vi "dataListenerMain.vi"() -> ()   [LabVIEW 2016]
doc: "Starts the Data Listener application. This method is the the same for each component."
uses:
  DataListenerThisComponent/DataListenerThisComponent.lvclass
  home/andres/ct_cmpuserevents/ComponentTemplateCore/ComponentModel/ComponentModel/DataListener/DataListener.lvclass
  CommandFactory/CommandFactory.lvclass
  home/andres/ct_cmpuserevents/ICommandFactory/ICommandFactory.lvclass
  PubSubDataEvent/PubSubDataEvent.lvclass
  ComponentTemplateCore/ComponentModel/ComponentModel/CommandEvent/CommandEvent.lvclass
  ComponentTemplateCore/ComponentModel/ComponentModel/MiddlewareProcessEvent/MiddlewareProcessEvent.lvclass
  ComponentTemplateCore/ComponentModel/ComponentModel/Rendezvous/Rendezvous.lvclass
  MiddlewareSALThisComponent/MiddlewareSALThisComponent.lvclass
  home/andres/ct_cmpuserevents/ComponentTemplateCore/ComponentModel/ComponentModel/Middleware/Middleware.lvclass
  MiddlewareSALThisComponent/ProgrammaticInitialization/ProgrammaticInitialization.lvclass
  DataListenerThisComponent/DataListenerThisComponent.lvclass/DataListenerThisComponent.ctl
  ComponentTemplateCore/ComponentModel/ComponentModel/Middleware/Middleware.lvclass/Middleware.ctl
  ComponentTemplateCore/ComponentModel/ComponentModel/DataListener/DataListener.lvclass/DataListener.ctl
  ComponentTemplateCore/ComponentModel/ComponentModel/DataListener/DataListener.lvclass
  ComponentTemplateCore/ComponentModel/ComponentModel/Middleware/Middleware.lvclass
  ComponentTemplateCore/ComponentModel/ComponentModel/ConfigurationFileReader/ConfigurationFileReader.lvclass
panel:
  out "error out":errorcluster
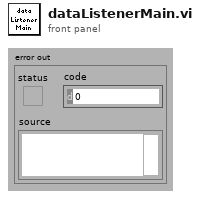
[diagram p1: front panel]
types:
  T1 = typedef "ConfigurationTypedefs.lvlib/SALVisSettings.ctl" = cluster{"SAL Vis Path":path, "Events":T2, "Telemetry":T3, "Subsystem":string, "Commands":T4}
  T2 = typedef "ProgrammaticInitialization.lvclass/evntsToSubscribeView.ctl" = string[]
  T3 = typedef "ProgrammaticInitialization.lvclass/tlmtryToSubscribeView.ctl" = string[]
  T4 = typedef "ProgrammaticInitialization.lvclass/cmdsToSubscribeDL.ctl" = string[]
  T5 = enum32{"Invalid", "Standard", "Closed", "Hidden", "Minimized", "Maximized"}
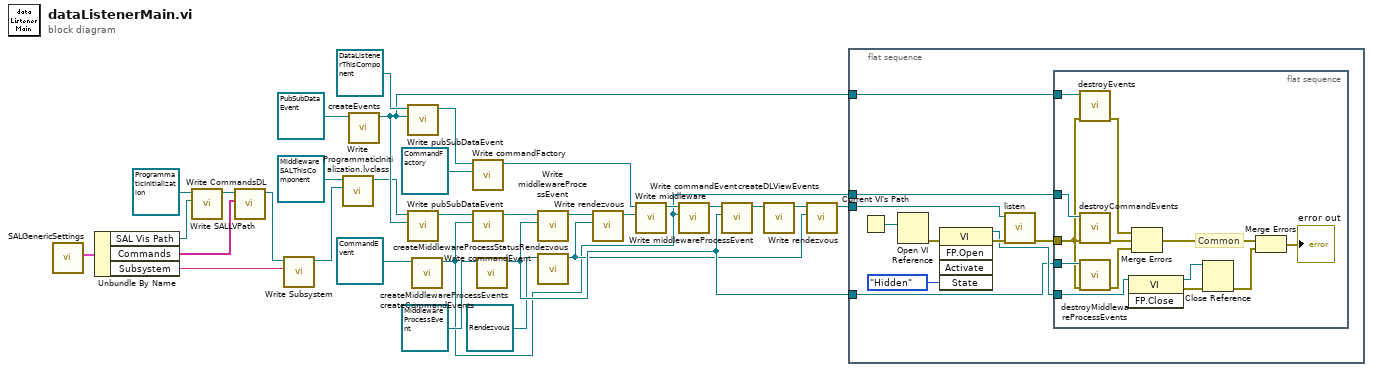
[diagram p0: block diagram]
diagram:
  n1 = call "SALGenericSettings.vi"() -> ("Generic SAL Definitions"=w4:T1)  [unwired: 9 in, 2 out]
  n2 = Unbundle By Name(w4) -> ("SAL Vis Path"=w1:path, "Commands"=w3:T4, "Subsystem"=w2:string)
  n3 = call-dynamic "Write SALLVPath.vi"("SALLVPath"=w1, "ProgrammaticInitialization in"=refnum<class "ProgrammaticInitialization.lvclass"> refnum ("ProgrammaticInitialization.lvclass")) -> ("ProgrammaticInitialization out"=w6:refnum<class "ProgrammaticInitialization.lvclass">)  [unwired: 8 in, 1 out]
  n4 = call-dynamic "Write CommandsDL.vi"("Commands"=w3, "ProgrammaticInitialization in"=w6) -> ("ProgrammaticInitialization out"=w5:refnum<class "ProgrammaticInitialization.lvclass">)  [unwired: 8 in, 1 out]
  n5 = call-dynamic "Write Subsystem.vi"("Subsystem"=w2, "ProgrammaticInitialization in"=w5) -> ("ProgrammaticInitialization out"=w8:refnum<class "ProgrammaticInitialization.lvclass">)  [unwired: 8 in, 1 out]
  n6 = call-dynamic "Write ProgrammaticInitialization.lvclass.vi"("ProgrammaticInitialization.lvclass"=w8, "MiddlewareSALThisComponent in"=refnum<class "MiddlewareSALThisComponent.lvclass"> refnum ("MiddlewareSALThisComponent.lvclass")) -> ("MiddlewareSALThisComponent out"=w10:refnum<class "MiddlewareSALThisComponent.lvclass">)  [unwired: 8 in, 1 out]
  n7 = call "createEvents.vi"("PubSubDataEvent in"=refnum<class "PubSubDataEvent.lvclass"> refnum ("PubSubDataEvent.lvclass")) -> ("PubSubDataEvent out"=w12:refnum<class "PubSubDataEvent.lvclass">)  [unwired: 9 in, 1 out]
  n8 = call "Write pubSubDataEvent.vi"("pubSubDataEvent"=w12, "DataListenerThisComponent in"=refnum<class "DataListenerThisComponent.lvclass"> refnum ("DataListenerThisComponent.lvclass")) -> ("DataListenerThisComponent out"=w22:refnum<class "DataListenerThisComponent.lvclass">)  [unwired: 9 in]
  n9 = call "Write pubSubDataEvent.vi"("pubSubDataEvent in"=w12, "MiddlewareSALThisComponent.lvclass in"=w10) -> ("MiddlewareSALThisComponent.lvclass out"=w11:refnum<class "MiddlewareSALThisComponent.lvclass">)  [unwired: 9 in]
  n10 = call "createCommandEvents.vi"("CommandEvent in"=refnum<class "CommandEvent.lvclass"> refnum ("CommandEvent.lvclass")) -> ("CommandEvent out"=w13:refnum<class "CommandEvent.lvclass">)  [unwired: 9 in, 1 out]
  n11 = call "Write commandFactory.vi"("commandFactory"=refnum<class "CommandFactory.lvclass"> refnum ("CommandFactory.lvclass"), "DataListenerThisComponent in"=w22) -> ("DataListenerThisComponent out"=w28:refnum<class "DataListenerThisComponent.lvclass">)  [unwired: 9 in]
  n12 = call "Write commandEvent.vi"("CommandEvent.lvclass"=w13, "Middleware in"=w11) -> ("Middleware out"=w24:refnum<class "MiddlewareSALThisComponent.lvclass">)  [unwired: 9 in]
  n13 = call "createMiddlewareProcessEvents.vi"("MiddlewareProcessEvent in"=refnum<class "MiddlewareProcessEvent.lvclass"> refnum ("MiddlewareProcessEvent.lvclass")) -> ("MiddlewareProcessEvent out"=w20:refnum<class "MiddlewareProcessEvent.lvclass">)  [unwired: 9 in, 1 out]
  n14 = call "Write middlewareProcessEvent.vi"("middlewareProcessEvent"=w20, "Middleware in"=w24) -> ("Middleware out"=w18:refnum<class "MiddlewareSALThisComponent.lvclass">)  [unwired: 9 in]
  n15 = call "createMiddlewareProcessStatusRendezvous.vi"("Rendezvous in"=refnum<class "Rendezvous.lvclass"> refnum ("Rendezvous.lvclass")) -> ("Rendezvous out"=w14:refnum<class "Rendezvous.lvclass">)  [unwired: 9 in, 1 out]
  n16 = call "Write rendezvous.vi"("Rendezvous.lvclass"=w14, "Middleware in"=w18) -> ("Middleware out"=w17:refnum<class "MiddlewareSALThisComponent.lvclass">)  [unwired: 9 in]
  n17 = call "Write middleware.vi"("middleware"=w17, "DataListener in"=w28) -> ("DataListener out"=w26:refnum<class "DataListenerThisComponent.lvclass">)  [unwired: 9 in]
  n18 = call "Write commandEvent.vi"("commandEvent"=w13, "DataListener in"=w26) -> ("DataListener out"=w23:refnum<class "DataListenerThisComponent.lvclass">)  [unwired: 9 in]
  n19 = call "Write middlewareProcessEvent.vi"("middlewareProcessEvent"=w20, "DataListener in"=w23) -> ("DataListener out"=w21:refnum<class "DataListenerThisComponent.lvclass">)  [unwired: 9 in]
  n20 = call "createDLViewEvents.vi"("DataListener in"=w21) -> ("DataListener out"=w16:refnum<class "DataListenerThisComponent.lvclass">)  [unwired: 9 in, 1 out]
  n21 = call "Write rendezvous.vi"("Rendezvous.lvclass"=w14, "DataListener in"=w16) -> ("DataListener out"=w15:refnum<class "DataListenerThisComponent.lvclass">)  [unwired: 9 in]
  n22 = flat-sequence {
    tunnel: w15 -> [w36]
    tunnel: w12 -> [w34]
    tunnel: w13 -> [w33]
    tunnel: w20 -> [w32]
    frame #0 {
      n23 = Current VI's Path() -> (path=w37:path)
      n24 = Open VI Reference(vi path=w37) -> (error out=w38:errorcluster)  [unwired: 5 in, 1 out]
      n25 = invoke class="VI" method="FP.Open"(error in=w38, "State"=T5."Hidden") -> (reference out=w40:refnum<vi>, error out=w41:errorcluster)  [unwired: 3 in, 3 out]
      n26 = call-dynamic "listen.vi"("error in (no error)"=w41, "DataListener in"=w36) -> ("error out"=w35:errorcluster)  [unwired: 8 in, 1 out]
      n27 = flat-sequence {
        tunnel: w40 -> [w54]
        tunnel: w35 -> [w47]
        tunnel: w34 -> [w48]
        tunnel: w33 -> [w49]
        tunnel: w32 -> [w50]
        frame #0 {
          # "Common"
          n28 = call "destroyEvents.vi"("error in (no error)"=w47, "PubSubDataEvent in"=w48) -> ("error out"=w45:errorcluster)  [unwired: 8 in, 1 out]
          n29 = call "destroyCommandEvents.vi"("error in (no error)"=w47, "CommandEvent in"=w49) -> ("error out"=w44:errorcluster)  [unwired: 8 in, 1 out]
          n30 = call "destroyMiddlewareProcessEvents.vi"("error in (no error)"=w47, "MiddlewareProcessEvent in"=w50) -> ("error out"=w43:errorcluster)  [unwired: 8 in, 1 out]
          n31 = invoke class="VI" method="FP.Close"(reference=w54) -> (reference out=w52:refnum<vi>, error out=w53:errorcluster)  [unwired: 2 in, 1 out]
          n32 = Merge Errors(w45, w44, w43) -> (w42:errorcluster)
          n33 = Close Reference(reference=w52, error in (no error)=w53) -> (error out=w51:errorcluster)
          n34 = Merge Errors(w42, w51) -> (→"error out":errorcluster)
        }
      }
    }
  }
